vi "GOOP_LVClass_Item_OnCommand.vi"(10 "Command Tag":string, 11 "Object":u64) -> ()   [LabVIEW 2020]
uses:
  <resource>/Framework/Providers/Open_GDS/SubVIs/GOOP_ClassProviderClassType.ctl
  <resource>/Framework/Providers/Open_GDS/ClassProviders/Provider_BaseClassInterface/ClassWriter_class/ClassWriter.lvclass
  <resource>/Framework/Providers/Open_GDS/ClassProviders/Common/ScriptingFunctions/Scripting_ConnectorPanePatternType.ctl
  <resource>/Framework/Providers/Open_GDS/SubVIs/GOOP_UMLEditor_CallMainAction.ctl
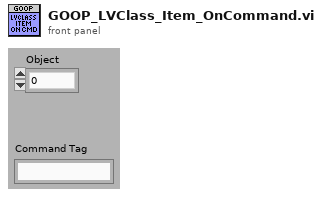
[diagram p1: front panel]
types:
  T1 = typedef "GOOP_ClassProviderClassType.ctl" = enum16{"ClassWriter", "ClassReader"}
  T2 = enum8{"No dynamic dispatch VIs", "Include nearest implementation", "Include all overrides"}
  T3 = typedef "GOOP_UMLEditor_CallMainAction.ctl" = enum16{"OpenUmlEditor", "ReverseEngineering:WholeProject", "ReverseEngineering:OneClass", "ReverseEngineering:OneVI", "ShowInStateDiagram:OneVI", "OpenUMLFile"}
  T4 = typedef "ClassWriter.lvclass/CreateMethodData.ctl" = cluster{"MethodName":string, "RelativeMethodPath":path, "MethodDescription":string, "Scope/Visibility":T5, "MethodTemplateName":string, "IconOut":u8[][], "RelativeProjectClassPath":string, "OpenViAfterCreation":bool, "DynamicDispatchVi":bool, "ExtraCreateParameters":variant, "MustOverride":bool, "MustCallParent":bool, "IconDetails":T6, "AF-Option":variant, "TemplatePath":path}
  T5 = typedef "GOOP300_MethodScopeType.ctl" = enum16{"Use Parent Folder Scope", "Public", "Protected", "Private", "Community"}
  T6 = typedef "ClassWriterNative.lvclass/IconDetails.ctl" = cluster{"IconSize":T7, "ImageRows(32)":i32, "ConnectorPaneHeight":i32[]}
  T7 = typedef "ClassWriterNative.lvclass/IconSize.ctl" = enum16{"Full", "1 c-term high", "2 c-term high", "3 c-term high"}
  T8 = typedef "AddDesignPatternData.ctl" = cluster{"Type":string, "ID":string, "Version":string, "VIPath":path, "Name":string, "Data":variant}
  T9 = typedef "ClassWriter.lvclass/CreateClassData.ctl" = cluster{"ClassName":string, "ClassFolder":path, "ClassDescription":string, "ClassTemplateOptions":string, "BaseClass(ProjectStringPath or LvClassFilePath)":variant, "ExtraCreateParameters":variant, "FolderSuffix":string}
  T10 = typedef "ClassWriter.lvclass/InterfacesToImplement.ctl" = cluster{"InterfacePath":path[], "CreateMethods":bool, "MethodsPerInterface(Empty=>All)":cluster{"Methods":string[]}[]}
  T11 = typedef "Scripting_ConnectorPanePatternType.ctl" = u16
  T12 = typedef "GDSLvCLass_ClassSettingsType.ctl" = cluster{"ClassProviderName":string, "ClassTemplateUsed":string, "ClassTemplateVersion":string, "ClassDescription":string, "PlugIns":T13[], "ConnectorPanePattern":string}
  T13 = typedef "GDSLvClass_PlugIn.ctl" = cluster{"Type":T14, "ID":string, "Version":string, "Path":path, "Name":string, "Data":variant}
  T14 = typedef "GDSLvClass_PlugInTypes.ctl" = enum16{"DesignPattern", "MethodTypes"}
  T15 = enum32{"invalid scope", "public", "private", "protected", "community"}
  T16 = typedef "ItemRef.ctl" = u64
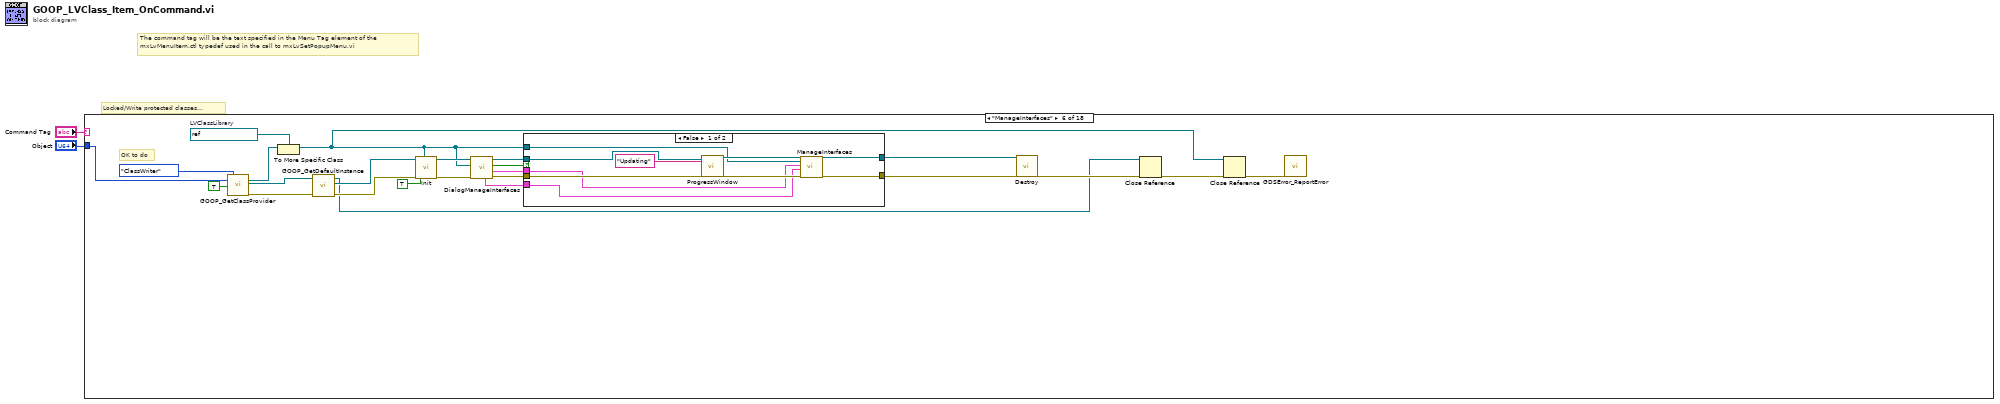
[diagram p0: block diagram]
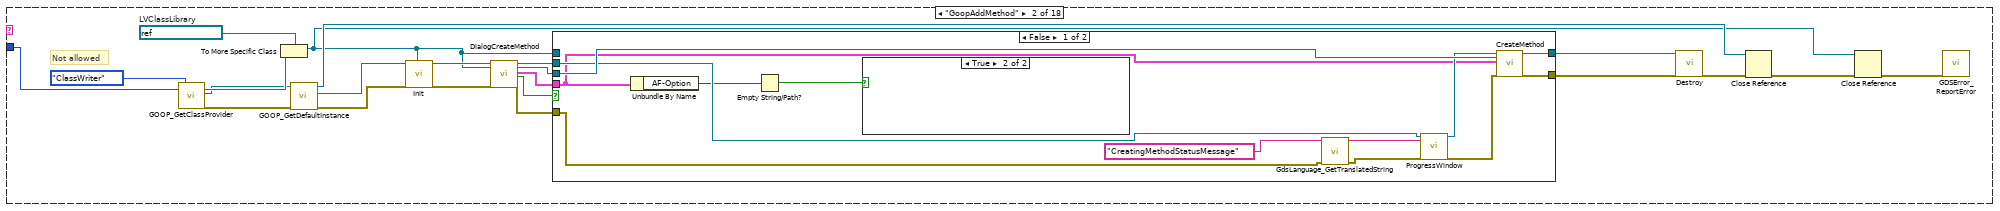
[diagram p3: hidden frame]
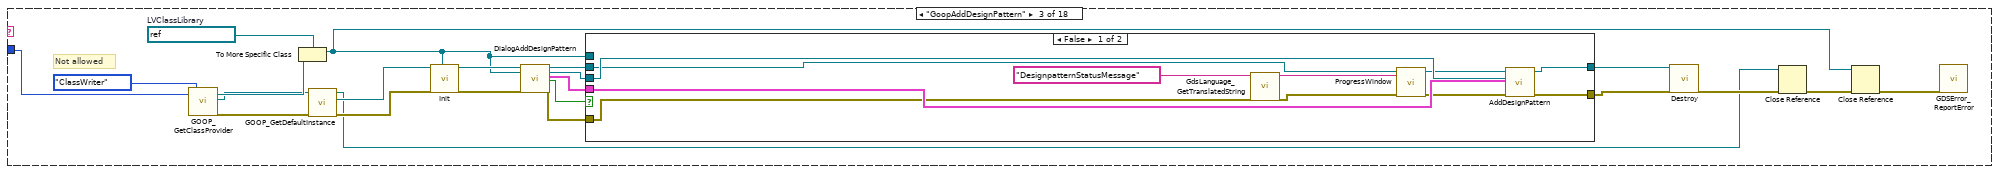
[diagram p6: hidden frame]
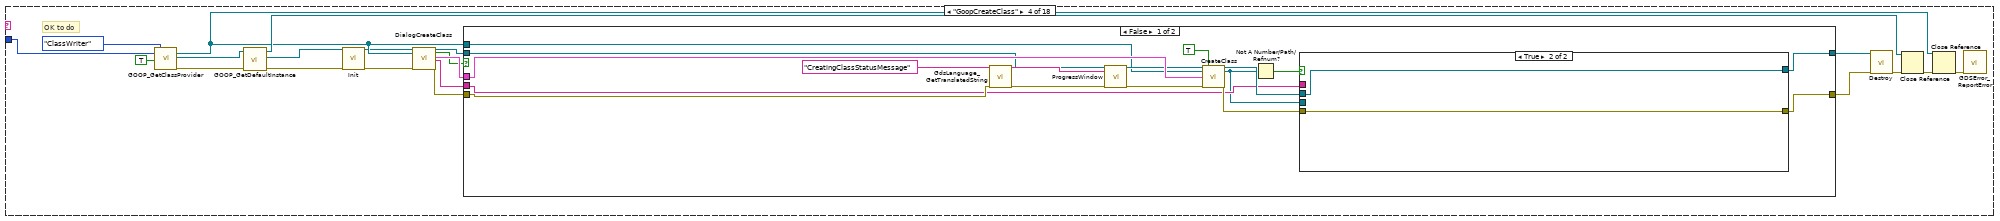
[diagram p8: hidden frame]
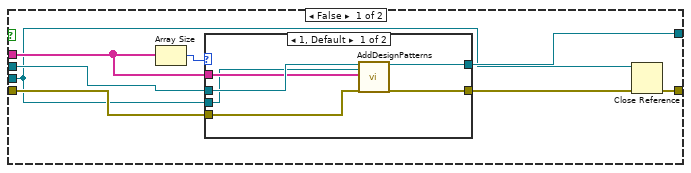
[diagram p9: hidden frame]
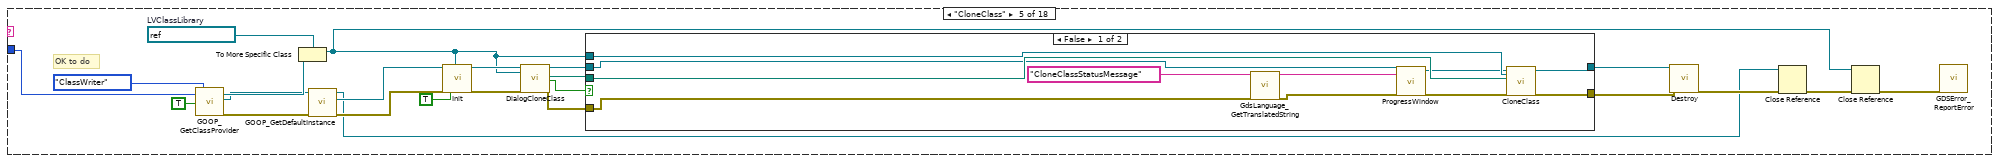
[diagram p12: hidden frame]
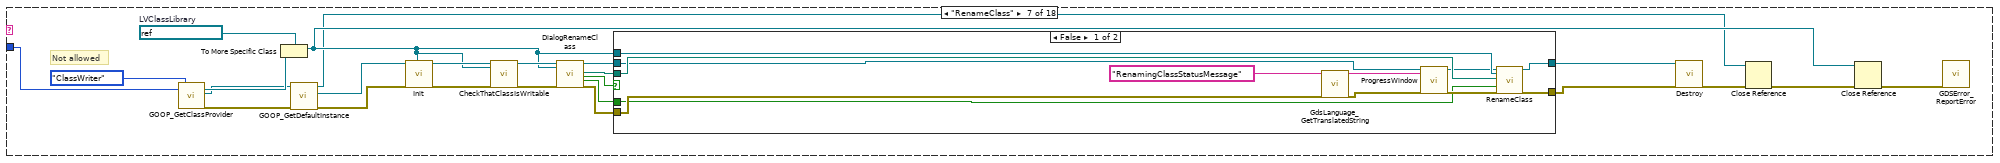
[diagram p15: hidden frame]
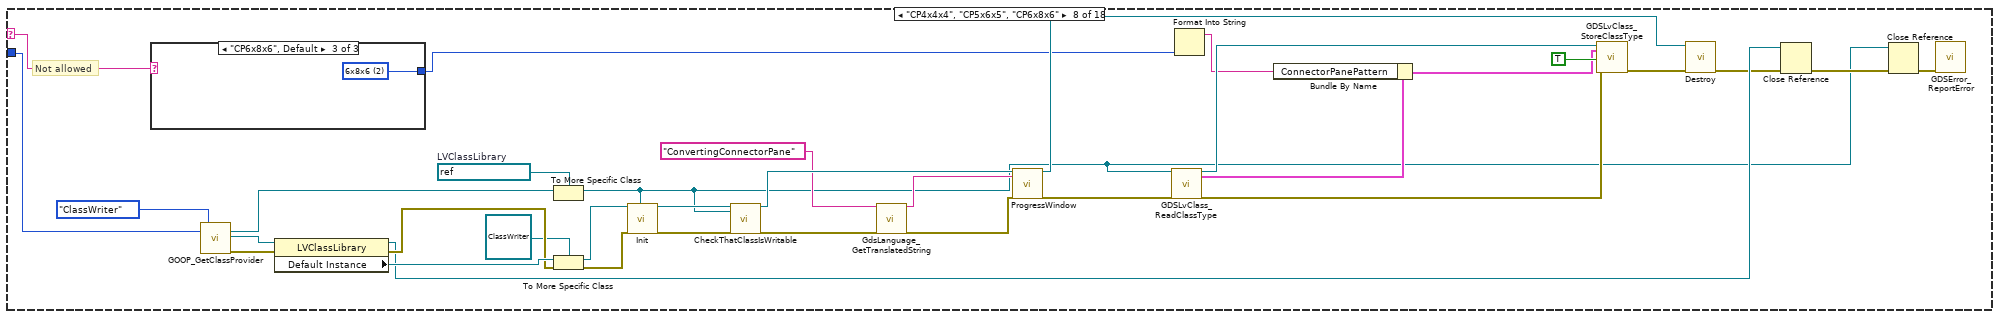
[diagram p17: hidden frame]
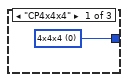
[diagram p18: hidden frame]
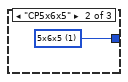
[diagram p19: hidden frame]
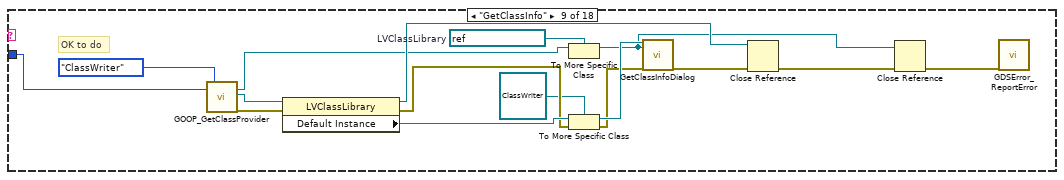
[diagram p20: hidden frame]
diagram:
  # "Locked/Write protected classes..."
  # "The command tag will be the text specified in the Menu Tag element of the \nmxLvMenuItem.ctl typedef used in the call to mxLvSetPopupMenu.vi"
  n1 = case shown="\"ManageInterfaces\"" "Command Tag" {
    selector: "Command Tag" -> [_ _ _ _ _ _ _ w243 _ _ _ _ _ _ w433 _ _ _]
    tunnel: "Object" -> [_ w24 w61 w95 w142 w185 w217 w263 w295 w296 w317 w324 w362 w381 w434 w463 w480 w527]
    frame "False" {
    }
    frame "GoopAddMethod" {
      w16 = refnum<vi> refnum  # LVClassLibrary
      # "Not allowed"
      n2 = call <resource>:"GOOP_GetClassProvider.vi"("New Item Parent/Object"=w24, "ProviderClassType"=GOOP_ClassProviderClassType."ClassWriter") -> ("ProjectItem"=w17:refnum<vi>, "LVClass.Open"=w5:refnum<vi>, "error out"=w4:errorcluster)  [unwired: 15 in]
      n3 = To More Specific Class(target class=w16, reference=w17) -> (specific class reference=w3:refnum<vi>)  [unwired: 1 in, 1 out]
      n4 = call <resource>:"GOOP_GetDefaultInstance.vi"("error in"=w4, "LVClassIn"=w5) -> ("error out"=w8:errorcluster, "ClassWriter.lvclass"=w7:refnum<class "ClassWriter.lvclass">, "LVClassOut"=w6:refnum<vi>)  [unwired: 7 in]
      n5 = call-dynamic "Init.vi"("ClassWriter in"=w7, "error in (no error)"=w8, "LVClassLibrary Refnum"=w3) -> ("ClassWriter out"=w9:refnum<class "ClassWriter.lvclass">, "error out"=w10:errorcluster)  [unwired: 15 in]
      n6 = call-dynamic "DialogCreateMethod.vi"("ClassWriter in"=w9, "ClassItemRefIn"=w3, "error in (no error)"=w10) -> ("ClassWriter out"=w20:refnum<class "ClassWriter.lvclass">, "ClassItemRefOut"=w19:refnum<vi>, "CreateMethodData"=w15:T4, "Cancelled"=w14:bool, "error out"=w18:errorcluster)  [unwired: 12 in]
      n7 = case shown="False" w14 {
        tunnel: w20 -> [w30 w38]
        tunnel: w19 -> [w37 _]
        tunnel: w18 -> [w32 w39]
        tunnel: w3 -> [_ _]
        tunnel: [w36 w39] -> w13
        tunnel: w15 -> [w27 _]
        tunnel: [w28 w38] -> w12
        frame False {
          n8 = Unbundle By Name(w27) -> ("AF-Option"=w26:variant)
          n9 = Empty String/Path?(string/path=w26) -> (empty?=w25:bool)
          n10 = case shown="True" w25 {
            frame False {
            }
            frame True {
            }
          }
          n11 = call <resource>:"GdsLanguage_GetTranslatedString.vi"("StringID(s)"="CreatingMethodStatusMessage" ("Message(Exit)"), "error in (no error)"=w32) -> ("FirstStringOut"=w35:string, "error out"=w34:errorcluster)  [unwired: 14 in, 2 out]
          n12 = call-dynamic "ProgressWindow.vi"("ClassWriter in"=w30, "Message(Exit)"=w35, "error in (no error)"=w34) -> ("ClassWriter out"=w29:refnum<class "ClassWriter.lvclass">, "error out"=w31:errorcluster)  [unwired: 15 in]
          n13 = call-dynamic "CreateMethod.vi"("ClassWriter.lvclass"=w29, "ClassItemRefIn"=w37, "CreateMethodData"=w27, "error in (no error)"=w31) -> ("ClassWriter.lvclass"=w28:refnum<class "ClassWriter.lvclass">, "error out"=w36:errorcluster)  [unwired: 12 in, 2 out]
        }
        frame True {
        }
      }
      n14 = call-dynamic "Destroy.vi"("ClassWriter.lvclass"=w12, "error in (no error)"=w13) -> ("error out"=w11:errorcluster)  [unwired: 17 in]
      n15 = Close Reference(reference=w6, error in (no error)=w11) -> (error out=w23:errorcluster)
      n16 = Close Reference(reference=w3, error in (no error)=w23) -> (error out=w22:errorcluster)
      n17 = call <resource>:"GDSError_ReportError.vi"("error in (no error)"=w22) -> ()  [unwired: 18 in, 1 out]
    }
    frame "GoopAddDesignPattern" {
      w53 = refnum<vi> refnum  # LVClassLibrary
      # "Not allowed"
      n18 = call <resource>:"GOOP_GetClassProvider.vi"("New Item Parent/Object"=w61, "ProviderClassType"=GOOP_ClassProviderClassType."ClassWriter") -> ("ProjectItem"=w54:refnum<vi>, "LVClass.Open"=w42:refnum<vi>, "error out"=w41:errorcluster)  [unwired: 15 in]
      n19 = To More Specific Class(target class=w53, reference=w54) -> (specific class reference=w40:refnum<vi>)  [unwired: 1 in, 1 out]
      n20 = call <resource>:"GOOP_GetDefaultInstance.vi"("error in"=w41, "LVClassIn"=w42) -> ("error out"=w45:errorcluster, "ClassWriter.lvclass"=w44:refnum<class "ClassWriter.lvclass">, "LVClassOut"=w43:refnum<vi>)  [unwired: 7 in]
      n21 = call-dynamic "Init.vi"("ClassWriter in"=w44, "error in (no error)"=w45, "LVClassLibrary Refnum"=w40) -> ("ClassWriter out"=w46:refnum<class "ClassWriter.lvclass">, "error out"=w47:errorcluster)  [unwired: 15 in]
      n22 = call-dynamic "DialogAddDesignPattern.vi"("ClassWriter in"=w46, "ClassItemRefIn"=w40, "error in (no error)"=w47) -> ("ClassWriter out"=w57:refnum<class "ClassWriter.lvclass">, "ClassItemRefOut"=w56:refnum<vi>, "CreateMethodData"=w52:T8, "Cancelled"=w51:bool, "error out"=w55:errorcluster)  [unwired: 12 in]
      n23 = case shown="False" w51 {
        tunnel: w57 -> [w64 w73]
        tunnel: w56 -> [w72 _]
        tunnel: w55 -> [w66 w74]
        tunnel: w40 -> [_ _]
        tunnel: [w70 w74] -> w50
        tunnel: w52 -> [w71 _]
        tunnel: [w62 w73] -> w49
        frame False {
          n24 = call <resource>:"GdsLanguage_GetTranslatedString.vi"("StringID(s)"="DesignpatternStatusMessage" ("Message(Exit)"), "error in (no error)"=w66) -> ("FirstStringOut"=w69:string, "error out"=w68:errorcluster)  [unwired: 14 in, 2 out]
          n25 = call-dynamic "ProgressWindow.vi"("ClassWriter in"=w64, "Message(Exit)"=w69, "error in (no error)"=w68) -> ("ClassWriter out"=w63:refnum<class "ClassWriter.lvclass">, "error out"=w65:errorcluster)  [unwired: 15 in]
          n26 = call-dynamic "AddDesignPattern.vi"("ClassWriter.lvclass"=w63, "ClassItemRefIn"=w72, "AddDesignPatternData"=w71, "error in (no error)"=w65) -> ("ClassWriter.lvclass"=w62:refnum<class "ClassWriter.lvclass">, "error out"=w70:errorcluster)  [unwired: 13 in, 1 out]
        }
        frame True {
        }
      }
      n27 = call-dynamic "Destroy.vi"("ClassWriter.lvclass"=w49, "error in (no error)"=w50) -> ("error out"=w48:errorcluster)  [unwired: 17 in]
      n28 = Close Reference(reference=w43, error in (no error)=w48) -> (error out=w60:errorcluster)
      n29 = Close Reference(reference=w40, error in (no error)=w60) -> (error out=w59:errorcluster)
      n30 = call <resource>:"GDSError_ReportError.vi"("error in (no error)"=w59) -> ()  [unwired: 18 in, 1 out]
    }
    frame "GoopCreateClass" {
      # "OK to do"
      n31 = call <resource>:"GOOP_GetClassProvider.vi"("New Item Parent/Object"=w95, "CreateClass"=TRUE, "ProviderClassType"=GOOP_ClassProviderClassType."ClassWriter") -> ("ProjectItem"=w84:refnum<vi>, "LVClass.Open"=w92:refnum<vi>, "error out"=w91:errorcluster)  [unwired: 14 in]
      n32 = call <resource>:"GOOP_GetDefaultInstance.vi"("error in"=w91, "LVClassIn"=w92) -> ("error out"=w76:errorcluster, "ClassWriter.lvclass"=w77:refnum<class "ClassWriter.lvclass">, "LVClassOut"=w87:refnum<vi>)  [unwired: 7 in]
      n33 = call-dynamic "Init.vi"("ClassWriter in"=w77, "error in (no error)"=w76) -> ("ClassWriter out"=w79:refnum<class "ClassWriter.lvclass">, "error out"=w78:errorcluster)  [unwired: 16 in]
      n34 = call-dynamic "DialogCreateClass.vi"("ClassWriter in"=w79, "ProjectItem Refnum"=w84, "error in (no error)"=w78) -> ("ClassWriter out"=w89:refnum<class "ClassWriter.lvclass">, "Cancelled"=w85:bool, "CreateClassData"=w86:T9, "DesignPatternsToAddAfterCreation"=w75:string[], "error out"=w88:errorcluster)  [unwired: 10 in, 2 out]
      n35 = case shown="False" w85 {
        tunnel: w89 -> [w107 w131]
        tunnel: w88 -> [w108 w132]
        tunnel: w84 -> [w100 _]
        tunnel: [w98 w132] -> w83
        tunnel: w86 -> [w112 _]
        tunnel: [w102 w131] -> w81
        tunnel: w75 -> [w101 _]
        frame False {
          n36 = call <resource>:"GdsLanguage_GetTranslatedString.vi"("StringID(s)"="CreatingClassStatusMessage" ("Message(Exit)"), "error in (no error)"=w108) -> ("FirstStringOut"=w109:string, "error out"=w110:errorcluster)  [unwired: 14 in, 2 out]
          n37 = call-dynamic "ProgressWindow.vi"("ClassWriter in"=w107, "Message(Exit)"=w109, "error in (no error)"=w110) -> ("ClassWriter out"=w106:refnum<class "ClassWriter.lvclass">, "error out"=w105:errorcluster)  [unwired: 15 in]
          n38 = call-dynamic "CreateClass.vi"("ClassWriter.lvclass"=w106, "ProjectTreePosition(String or Project Item Ref)"=w100, "CreateClassData"=w112, "error in (no error)"=w105, "KeepLvClassRefOpen(False)"=TRUE) -> ("ClassWriter.lvclass"=w104:refnum<class "ClassWriter.lvclass">, "LVClassLibraryRefnum"=w97:refnum<vi>, "error out"=w103:errorcluster)  [unwired: 11 in, 1 out]
          n39 = Not A Number/Path/Refnum?(number/path/refnum=w97) -> (NaN/Path/Refnum?=w96:bool)
          n40 = case shown="True" w96 {
            tunnel: w104 -> [w119 w130]
            tunnel: w103 -> [w118 w129]
            tunnel: [w117 w130] -> w102
            tunnel: w101 -> [w116 _]
            tunnel: [w114 w129] -> w98
            tunnel: w97 -> [w113 _]
            frame False {
              n41 = Array Size(array=w116) -> (size(s)=w120:i32)
              n42 = case shown="1, Default" w120 {
                tunnel: w119 -> [w126 w128]
                tunnel: w118 -> [w125 w127]
                tunnel: [w124 w127] -> w115
                tunnel: [w123 w128] -> w117
                tunnel: w116 -> [w122 _]
                tunnel: w113 -> [w121 _]
                frame 1, Default {
                  n43 = call-dynamic "AddDesignPatterns.vi"("ClassWriterNative"=w126, "ClassItemRefIn"=w121, "DesignPatterns"=w122, "error in (no error)"=w125) -> ("ClassWriterNative"=w123:refnum<class "ClassWriter.lvclass">, "error out"=w124:errorcluster)  [unwired: 12 in, 2 out]
                }
                frame 0 {
                }
              }
              n44 = Close Reference(reference=w113, error in (no error)=w115) -> (error out=w114:errorcluster)
            }
            frame True {
            }
          }
        }
        frame True {
        }
      }
      n45 = call-dynamic "Destroy.vi"("ClassWriter.lvclass"=w81, "error in (no error)"=w83) -> ("error out"=w82:errorcluster)  [unwired: 17 in]
      n46 = Close Reference(reference=w87, error in (no error)=w82) -> (error out=w94:errorcluster)
      n47 = Close Reference(reference=w84, error in (no error)=w94) -> (error out=w93:errorcluster)
      n48 = call <resource>:"GDSError_ReportError.vi"("error in (no error)"=w93) -> ()  [unwired: 18 in, 1 out]
    }
    frame "CloneClass" {
      w152 = refnum<vi> refnum  # LVClassLibrary
      # "OK to do"
      n49 = call <resource>:"GOOP_GetClassProvider.vi"("New Item Parent/Object"=w142, "CreateClass"=TRUE, "ProviderClassType"=GOOP_ClassProviderClassType."ClassWriter") -> ("ProjectItem"=w153:refnum<vi>, "LVClass.Open"=w139:refnum<vi>, "error out"=w140:errorcluster)  [unwired: 14 in]
      n50 = To More Specific Class(target class=w152, reference=w153) -> (specific class reference=w133:refnum<vi>)  [unwired: 1 in, 1 out]
      n51 = call <resource>:"GOOP_GetDefaultInstance.vi"("error in"=w140, "LVClassIn"=w139) -> ("error out"=w137:errorcluster, "ClassWriter.lvclass"=w138:refnum<class "ClassWriter.lvclass">, "LVClassOut"=w136:refnum<vi>)  [unwired: 7 in]
      n52 = call-dynamic "Init.vi"("ClassWriter in"=w138, "error in (no error)"=w137, "ClassFileMayBeReadOnly(False)"=TRUE, "LVClassLibrary Refnum"=w133) -> ("ClassWriter out"=w145:refnum<class "ClassWriter.lvclass">, "error out"=w144:errorcluster)  [unwired: 14 in]
      n53 = call-dynamic "DialogCloneClass.vi"("ClassWriter.lvclass"=w145, "ClassItemRefIn"=w133, "error in (no error)"=w144) -> ("ClassWriter.lvclassOut"=w150:refnum<class "ClassWriter.lvclass">, "NewClassPath"=w146:path, "Cancelled"=w147:bool, "error out"=w149:errorcluster)  [unwired: 12 in, 1 out]
      n54 = case shown="False" w147 {
        tunnel: w150 -> [w158 w167]
        tunnel: w149 -> [w159 w168]
        tunnel: [w163 w168] -> w148
        tunnel: w133 -> [w166 _]
        tunnel: w146 -> [w165 _]
        tunnel: [w164 w167] -> w143
        frame False {
          n55 = call <resource>:"GdsLanguage_GetTranslatedString.vi"("StringID(s)"="CloneClassStatusMessage" ("Message(Exit)"), "error in (no error)"=w159) -> ("FirstStringOut"=w160:string, "error out"=w161:errorcluster)  [unwired: 14 in, 2 out]
          n56 = call-dynamic "ProgressWindow.vi"("ClassWriter in"=w158, "Message(Exit)"=w160, "error in (no error)"=w161) -> ("ClassWriter out"=w157:refnum<class "ClassWriter.lvclass">, "error out"=w156:errorcluster)  [unwired: 15 in]
          n57 = call-dynamic "CloneClass.vi"("ClassWriter.lvclass"=w157, "ClassRef"=w166, "NewClassPath"=w165, "error in (no error)"=w156) -> ("ClassWriter.lvclass"=w164:refnum<class "ClassWriter.lvclass">, "error out"=w163:errorcluster)  [unwired: 13 in, 1 out]
        }
        frame True {
        }
      }
      n58 = call-dynamic "Destroy.vi"("ClassWriter.lvclass"=w143, "error in (no error)"=w148) -> ("error out"=w151:errorcluster)  [unwired: 17 in]
      n59 = Close Reference(reference=w136, error in (no error)=w151) -> (error out=w155:errorcluster)
      n60 = Close Reference(reference=w133, error in (no error)=w155) -> (error out=w141:errorcluster)
      n61 = call <resource>:"GDSError_ReportError.vi"("error in (no error)"=w141) -> ()  [unwired: 18 in, 1 out]
    }
    frame "ManageInterfaces" {
      w189 = refnum<vi> refnum  # LVClassLibrary
      # "OK to do"
      n62 = call <resource>:"GOOP_GetClassProvider.vi"("New Item Parent/Object"=w185, "CreateClass"=TRUE, "ProviderClassType"=GOOP_ClassProviderClassType."ClassWriter") -> ("ProjectItem"=w190:refnum<vi>, "LVClass.Open"=w182:refnum<vi>, "error out"=w183:errorcluster)  [unwired: 14 in]
      n63 = To More Specific Class(target class=w189, reference=w190) -> (specific class reference=w171:refnum<vi>)  [unwired: 1 in, 1 out]
      n64 = call <resource>:"GOOP_GetDefaultInstance.vi"("error in"=w183, "LVClassIn"=w182) -> ("error out"=w180:errorcluster, "ClassWriter.lvclass"=w181:refnum<class "ClassWriter.lvclass">, "LVClassOut"=w179:refnum<vi>)  [unwired: 7 in]
      n65 = call-dynamic "Init.vi"("ClassWriter in"=w181, "error in (no error)"=w180, "ClassFileMayBeReadOnly(False)"=TRUE, "LVClassLibrary Refnum"=w171) -> ("ClassWriter out"=w176:refnum<class "ClassWriter.lvclass">, "error out"=w175:errorcluster)  [unwired: 14 in]
      n66 = call-dynamic "DialogManageInterfaces.vi"("error in (no error)"=w175, "ClassItemRefIn"=w171, "ClassWriterIn"=w176) -> ("error out"=w173:errorcluster, "InterfaceToAdd"=w170:T10, "Cancelled"=w174:bool, "ClassWriterOut"=w172:refnum<class "ClassWriter.lvclass">, "InterfaceToRemove(CreateMethod=>RemoveMethods)"=w169:T10)  [unwired: 4 in]
      n67 = case shown="False" w174 {
        tunnel: w172 -> [w202 w203]
        tunnel: w173 -> [w200 w204]
        tunnel: [w197 w204] -> w187
        tunnel: w171 -> [w195 _]
        tunnel: [w196 w203] -> w186
        tunnel: w170 -> [w194 _]
        tunnel: w169 -> [w193 _]
        frame False {
          n68 = call-dynamic "ProgressWindow.vi"("ClassWriter in"=w202, "Message(Exit)"="Updating", "error in (no error)"=w200) -> ("ClassWriter out"=w199:refnum<class "ClassWriter.lvclass">, "error out"=w198:errorcluster)  [unwired: 15 in]
          n69 = call-dynamic "ManageInterfaces.vi"("ClassWriter.lvclass"=w199, "ClassRef"=w195, "InterfaceToAdd"=w194, "InterfaceToRemove(CreateMethod=>RemoveMethods)"=w193, "error in (no error)"=w198) -> ("ClassWriter.lvclass"=w196:refnum<class "ClassWriter.lvclass">, "error out"=w197:errorcluster)  [unwired: 13 in]
        }
        frame True {
        }
      }
      n70 = call-dynamic "Destroy.vi"("ClassWriter.lvclass"=w186, "error in (no error)"=w187) -> ("error out"=w188:errorcluster)  [unwired: 17 in]
      n71 = Close Reference(reference=w179, error in (no error)=w188) -> (error out=w192:errorcluster)
      n72 = Close Reference(reference=w171, error in (no error)=w192) -> (error out=w184:errorcluster)
      n73 = call <resource>:"GDSError_ReportError.vi"("error in (no error)"=w184) -> ()  [unwired: 18 in, 1 out]
    }
    frame "RenameClass" {
      w225 = refnum<vi> refnum  # LVClassLibrary
      # "Not allowed"
      n74 = call <resource>:"GOOP_GetClassProvider.vi"("New Item Parent/Object"=w217, "ProviderClassType"=GOOP_ClassProviderClassType."ClassWriter") -> ("ProjectItem"=w226:refnum<vi>, "LVClass.Open"=w208:refnum<vi>, "error out"=w209:errorcluster)  [unwired: 15 in]
      n75 = To More Specific Class(target class=w225, reference=w226) -> (specific class reference=w211:refnum<vi>)  [unwired: 1 in, 1 out]
      n76 = call <resource>:"GOOP_GetDefaultInstance.vi"("error in"=w209, "LVClassIn"=w208) -> ("error out"=w206:errorcluster, "ClassWriter.lvclass"=w207:refnum<class "ClassWriter.lvclass">, "LVClassOut"=w205:refnum<vi>)  [unwired: 7 in]
      n77 = call-dynamic "Init.vi"("ClassWriter in"=w207, "error in (no error)"=w206, "LVClassLibrary Refnum"=w211) -> ("ClassWriter out"=w215:refnum<class "ClassWriter.lvclass">, "error out"=w214:errorcluster)  [unwired: 15 in]
      n78 = call <resource>:"CheckThatClassIsWritable.vi"("ClassWriter in"=w215, "Library Refnum"=w211, "error in (no error)"=w214) -> ("ClassWriter out"=w213:refnum<class "ClassWriter.lvclass">, "error out"=w212:errorcluster)  [unwired: 15 in]
      n79 = call-dynamic "DialogRenameClass.vi"("ClassWriter.lvclass"=w213, "ClassItemRefIn"=w211, "error in (no error)"=w212) -> ("ClassWriter.lvclassOut"=w223:refnum<class "ClassWriter.lvclass">, "NewClassPath"=w219:path, "Cancelled"=w220:bool, "RelinkWholeProject"=w210:bool, "error out"=w222:errorcluster)  [unwired: 11 in, 1 out]
      n80 = case shown="False" w220 {
        tunnel: w223 -> [w236 w241]
        tunnel: w222 -> [w233 w242]
        tunnel: [w237 w242] -> w221
        tunnel: w211 -> [w240 _]
        tunnel: w219 -> [w239 _]
        tunnel: [w238 w241] -> w218
        tunnel: w210 -> [w229 _]
        frame False {
          n81 = call <resource>:"GdsLanguage_GetTranslatedString.vi"("StringID(s)"="RenamingClassStatusMessage" ("Message(Exit)"), "error in (no error)"=w233) -> ("FirstStringOut"=w230:string, "error out"=w232:errorcluster)  [unwired: 14 in, 2 out]
          n82 = call-dynamic "ProgressWindow.vi"("ClassWriter in"=w236, "Message(Exit)"=w230, "error in (no error)"=w232) -> ("ClassWriter out"=w235:refnum<class "ClassWriter.lvclass">, "error out"=w234:errorcluster)  [unwired: 15 in]
          n83 = call-dynamic "RenameClass.vi"("ClassWriter.lvclass"=w235, "ClassRef"=w240, "NewClassPath"=w239, "RelinkWholeProject"=w229, "error in (no error)"=w234) -> ("ClassWriter.lvclass"=w238:refnum<class "ClassWriter.lvclass">, "error out"=w237:errorcluster)  [unwired: 13 in]
        }
        frame True {
        }
      }
      n84 = call-dynamic "Destroy.vi"("ClassWriter.lvclass"=w218, "error in (no error)"=w221) -> ("error out"=w224:errorcluster)  [unwired: 17 in]
      n85 = Close Reference(reference=w205, error in (no error)=w224) -> (error out=w228:errorcluster)
      n86 = Close Reference(reference=w211, error in (no error)=w228) -> (error out=w216:errorcluster)
      n87 = call <resource>:"GDSError_ReportError.vi"("error in (no error)"=w216) -> ()  [unwired: 18 in, 1 out]
    }
    frame "CP4x4x4", "CP5x6x5", "CP6x8x6" {
      w269 = refnum<vi> refnum  # LVClassLibrary
      # "Not allowed"
      n88 = case shown="\"CP6x8x6\", Default" w243 {
        tunnel: [w277 w278 w279] -> w245
        frame "CP4x4x4" {
          w277 = T11 0 items=["4x4x4", "5x6x5", "6x8x6"] ("Pattern")
        }
        frame "CP5x6x5" {
          w278 = T11 1 items=["4x4x4", "5x6x5", "6x8x6"] ("Pattern")
        }
        frame "CP6x8x6", Default {
          w279 = T11 2 items=["4x4x4", "5x6x5", "6x8x6"] ("Pattern")
        }
      }
      n89 = call <resource>:"GOOP_GetClassProvider.vi"("New Item Parent/Object"=w263, "ProviderClassType"=GOOP_ClassProviderClassType."ClassWriter") -> ("ProjectItem"=w270:refnum<vi>, "LVClass.Open"=w268:refnum<vi>, "error out"=w273:errorcluster)  [unwired: 15 in]
      n90 = property class="LVClassLibrary"(reference=w268, error in=w273) -> (reference out=w271:refnum<vi>, error out=w275:errorcluster, "Default Instance"=w276:refnum<class>)
      n91 = To More Specific Class(target class=w269, reference=w270) -> (specific class reference=w249:refnum<vi>)  [unwired: 1 in, 1 out]
      n92 = To More Specific Class(target class=refnum<class "ClassWriter.lvclass"> refnum ("ClassWriter.lvclass"), reference=w276, error in=w275) -> (specific class reference=w264:refnum<class "ClassWriter.lvclass">, error out=w265:errorcluster)
      n93 = call-dynamic "Init.vi"("ClassWriter in"=w264, "error in (no error)"=w265, "LVClassLibrary Refnum"=w249) -> ("ClassWriter out"=w261:refnum<class "ClassWriter.lvclass">, "error out"=w260:errorcluster)  [unwired: 15 in]
      n94 = call <resource>:"CheckThatClassIsWritable.vi"("ClassWriter in"=w261, "Library Refnum"=w249, "error in (no error)"=w260) -> ("ClassWriter out"=w258:refnum<class "ClassWriter.lvclass">, "error out"=w259:errorcluster)  [unwired: 15 in]
      n95 = call <resource>:"GdsLanguage_GetTranslatedString.vi"("StringID(s)"="ConvertingConnectorPane" ("Message(Exit)"), "error in (no error)"=w259) -> ("FirstStringOut"=w255:string, "error out"=w257:errorcluster)  [unwired: 14 in, 2 out]
      n96 = call-dynamic "ProgressWindow.vi"("ClassWriter in"=w258, "Message(Exit)"=w255, "error in (no error)"=w257) -> ("ClassWriter out"=w254:refnum<class "ClassWriter.lvclass">, "error out"=w253:errorcluster)  [unwired: 15 in]
      n97 = call <resource>:"GDSLvClass_ReadClassType.vi"("Class Refnum In"=w249, "error in (no error)"=w253) -> ("Class Refnum Out"=w252:refnum<vi>, "ClassSettings"=w251:T12, "error out"=w250:errorcluster)  [unwired: 15 in]
      n98 = Format Into String(w245) -> (resulting string=w244:string)  [unwired: 3 in, 1 out]
      n99 = Bundle By Name(cluster=w251, "ConnectorPanePattern"=w244) -> (w246:T12)
      n100 = call <resource>:"GDSLvClass_StoreClassType.vi"("Class Refnum In"=w252, "ClassSettings"=w246, "CheckAndFixConnectorPaneType(False)"=TRUE, "error in (no error)"=w250) -> ("error out"=w248:errorcluster)  [unwired: 14 in, 1 out]
      n101 = call-dynamic "Destroy.vi"("ClassWriter.lvclass"=w254, "error in (no error)"=w248) -> ("error out"=w267:errorcluster)  [unwired: 17 in]
      n102 = Close Reference(reference=w271, error in (no error)=w267) -> (error out=w274:errorcluster)
      n103 = Close Reference(reference=w249, error in (no error)=w274) -> (error out=w262:errorcluster)
      n104 = call <resource>:"GDSError_ReportError.vi"("error in (no error)"=w262) -> ()  [unwired: 18 in, 1 out]
    }
    frame "GetClassInfo" {
      w284 = refnum<vi> refnum  # LVClassLibrary
      # "OK to do"
      n105 = call <resource>:"GOOP_GetClassProvider.vi"("New Item Parent/Object"=w295, "ProviderClassType"=GOOP_ClassProviderClassType."ClassWriter") -> ("ProjectItem"=w285:refnum<vi>, "LVClass.Open"=w290:refnum<vi>, "error out"=w289:errorcluster)  [unwired: 15 in]
      n106 = property class="LVClassLibrary"(reference=w290, error in=w289) -> (reference out=w287:refnum<vi>, error out=w293:errorcluster, "Default Instance"=w294:refnum<class>)
      n107 = To More Specific Class(target class=w284, reference=w285) -> (specific class reference=w280:refnum<vi>)  [unwired: 1 in, 1 out]
      n108 = To More Specific Class(target class=refnum<class "ClassWriter.lvclass"> refnum ("ClassWriter.lvclass"), reference=w294, error in=w293) -> (specific class reference=w283:refnum<class "ClassWriter.lvclass">, error out=w282:errorcluster)
      n109 = call-dynamic "GetClassInfoDialog.vi"("ClassWriter in"=w283, "ClassItemRefIn"=w280, "error in (no error)"=w282) -> ("error out"=w281:errorcluster)  [unwired: 15 in, 1 out]
      n110 = Close Reference(reference=w287, error in (no error)=w281) -> (error out=w292:errorcluster)
      n111 = Close Reference(reference=w280, error in (no error)=w292) -> (error out=w291:errorcluster)
      n112 = call <resource>:"GDSError_ReportError.vi"("error in (no error)"=w291) -> ()  [unwired: 18 in, 1 out]
    }
    frame "DebugClass" {
      w305 = refnum<vi> refnum  # LVClassLibrary
      # "OK to do"
      n113 = call <resource>:"GOOP_GetClassProvider.vi"("New Item Parent/Object"=w296, "ProviderClassType"=GOOP_ClassProviderClassType."ClassWriter") -> ("ProjectItem"=w306:refnum<vi>, "LVClass.Open"=w304:refnum<vi>, "error out"=w297:errorcluster)  [unwired: 15 in]
      n114 = To More Specific Class(target class=w305, reference=w306, error in=w297) -> (specific class reference=w303:refnum<vi>, error out=w298:errorcluster)
      n115 = property class="LVClassLibrary"(reference=w303, error in=w298) -> (reference out=w302:refnum<vi>, error out=w299:errorcluster, "Name"=w301:string)
      n116 = call <resource>:"GOOP_StartObjectDebugger.vi"("ClassToOpen"=w301, "error in (no error)"=w299) -> ("error out"=w300:errorcluster)  [unwired: 17 in]
      n117 = Close Reference(reference=w304, error in (no error)=w300) -> (error out=w309:errorcluster)
      n118 = Close Reference(reference=w302, error in (no error)=w309) -> (error out=w308:errorcluster)
      n119 = call <resource>:"GDSError_ReportError.vi"("error in (no error)"=w308) -> ()  [unwired: 18 in, 1 out]
    }
    frame "GoopEditClassIcon" {
      w318 = refnum<vi> refnum  # LVClassLibrary
      # "Not allowed"
      n120 = call <resource>:"mxLvGetItemRef.vi"("Item"=w317) -> ("Item Refnum"=w316:refnum<vi>, "error out"=w311:errorcluster)  [unwired: 1 in, 1 out]
      n121 = To More Specific Class(target class=w318, reference=w316) -> (specific class reference=w310:refnum<vi>)  [unwired: 1 in, 1 out]
      n122 = call <resource>:"GOOP_CheckClassState.vi"("error in"=w311, "Library Refnum"=w310) -> ("error out"=w312:errorcluster)  [unwired: 9 in]
      n123 = call <resource>:"CheckThatClassIsWritable.vi"("Library Refnum"=w310, "error in (no error)"=w312) -> ("error out"=w313:errorcluster)  [unwired: 16 in, 1 out]
      n124 = call <resource>:"GDSLvIcon_DialogUpdateClass.vi"("ClassPath(FilePath/ProjectTreePath/LvCLassRef)"=w310, "error in (no error)"=w313) -> ("error out"=w315:errorcluster)  [unwired: 14 in, 3 out]
      n125 = Close Reference(reference=w310, error in (no error)=w315) -> (error out=w314:errorcluster)
      n126 = call <resource>:"GDSError_ReportError.vi"("error in (no error)"=w314) -> ()  [unwired: 18 in, 1 out]
    }
    frame "ClassTool" {
      w325 = refnum<vi> refnum  # LVClassLibrary
      # "Not allowed"
      n127 = call <resource>:"mxLvGetItemRef.vi"("Item"=w324) -> ("Item Refnum"=w323:refnum<vi>, "error out"=w321:errorcluster)  [unwired: 1 in, 1 out]
      n128 = To More Specific Class(target class=w325, reference=w323) -> (specific class reference=w320:refnum<vi>)  [unwired: 1 in, 1 out]
      n129 = call <resource>:"GOOP_ClassTool.vi"("ClassRef"=w320, "Error In"=w321) -> ("Error Out"=w319:errorcluster)  [unwired: 17 in]
      n130 = Close Reference(reference=w320, error in (no error)=w319) -> (error out=w322:errorcluster)
      n131 = call <resource>:"GDSError_ReportError.vi"("error in (no error)"=w322) -> ()  [unwired: 18 in, 1 out]
    }
    frame "UpdateMessageClass" {
      w363 = refnum<vi> refnum  # LVClassLibrary
      # "From Message Class Ref\nGet Actor method"
      # "Not allowed"
      n132 = call <resource>:"mxLvGetItemRef.vi"("Item"=w362) -> ("Item Refnum"=w361:refnum<vi>, "error out"=w337:errorcluster)  [unwired: 1 in, 1 out]
      n133 = call-dynamic "Init.vi"("ClassWriter in"=refnum<class "ClassWriter.lvclass"> refnum, "error in (no error)"=w337) -> ("ClassWriter out"=w331:refnum<class "ClassWriter.lvclass">, "error out"=w334:errorcluster)  [unwired: 16 in]
      n134 = call <resource>:"GdsLanguage_GetTranslatedString.vi"("StringID(s)"="UpdateMessageClass" ("Message(Exit)"), "error in (no error)"=w334) -> ("FirstStringOut"=w335:string, "error out"=w333:errorcluster)  [unwired: 14 in, 2 out]
      n135 = disable-structure shown="Enabled" {
        disable-tunnel: w335 -> [w368 _]
        disable-tunnel: [w367 w370] -> w328
        disable-tunnel: w333 -> [w366 w370]
        disable-tunnel: w331 -> [w365 w369]
        disable-tunnel: [w364 w369] -> w330
        frame Enabled {
          n136 = call-dynamic "ProgressWindow.vi"("ClassWriter in"=w365, "Message(Exit)"=w368, "error in (no error)"=w366) -> ("ClassWriter out"=w364:refnum<class "ClassWriter.lvclass">, "error out"=w367:errorcluster)  [unwired: 15 in]
        }
        frame Disabled {
        }
      }
      n137 = To More Specific Class(target class=w363, reference=w361) -> (specific class reference=w327:refnum<vi>)  [unwired: 1 in, 1 out]
      n138 = property class="LVClassLibrary"(reference=w327, error in=w328) -> (error out=w359:errorcluster, "Project"=w358:refnum<vi>, "Path"=w355:path)  [unwired: 1 out]
      n139 = property class="Project"(reference=w358, error in=w359) -> (error out=w348:errorcluster, "App Ref"=w357:refnum<vi>)  [unwired: 1 out]
      n140 = invoke class="LVClassLibrary" method="Get All Descendents"(reference=w327, error in=w348, "Type"="VI") -> (error out=w350:errorcluster, "All Descendents"=w342:refnum<vi>[])  [unwired: 4 in, 5 out]
      n141 = for {
        tunnel: w342 -> [w378] mode=indexing
        tunnel: [w374] -> w352
        shift-right: [w373] -> w351
        shift-left: w350 -> [w372]
        stop <- w371 stop-if-true
        n142 = property class="ProjectItem"(reference=w378, error in=w372) -> (reference out=w374:refnum<vi>, error out=w373:errorcluster, "Name"=w377:string)
        n143 = To Lower Case(string=w377) -> (all lower case string=w376:string)
        n144 = Equal?(x=w376, y="do.vi") -> (x = y?=w371:bool)
      }
      n145 = Strip Path(path=w355) -> (stripped path=w354:path)  [unwired: 1 out]
      n146 = property class="ProjectItem"(reference=w352, error in=w351) -> (error out=w346:errorcluster, "Reference"=w349:refnum<vi>)  [unwired: 1 out]
      n147 = invoke class="VI" method="Get VI Dependencies"(reference=w349, error in=w346, "Dynamic Dispatching?"=T2."Include nearest implementation") -> (reference out=w344:refnum<vi>, error out=w345:errorcluster, "Dependency Paths"=w341:path[])  [unwired: 16 in, 16 out]
      n148 = Close Reference(reference=w344, error in (no error)=w345) -> (error out=w343:errorcluster)
      n149 = Index Array(array=w341) -> (element=w340:path)  [unwired: 1 in]
      n150 = Close Reference(reference=w342, error in (no error)=w343) -> (error out=w339:errorcluster)
      n151 = call <resource>:"MM.vi"("AppInst"=w357, "ActorMethod"=w340, "ActorClassItemRef(Don't Delete)"=refnum<vi> refnum, "OnlyUpdate(if needed,False)"=TRUE ("OnlyUpdate(if needed)"), "Destination Path"=w354, "error in"=w339) -> ("error out"=w338:errorcluster)  [unwired: 13 in]
      n152 = Close Reference(reference=w327, error in (no error)=w338) -> (error out=w360:errorcluster)
      n153 = call <resource>:"GDSError_ReportError.vi"("error in (no error)"=w360) -> ("error out"=w332:errorcluster)  [unwired: 18 in]
      n154 = call-dynamic "Destroy.vi"("ClassWriter.lvclass"=w330, "error in (no error)"=w332) -> ()  [unwired: 17 in, 1 out]
    }
    frame "UpdateMessageClasses" {
      w406 = refnum<vi> refnum  # LVClassLibrary
      # "From Message Class Ref\nGet Actor method"
      n155 = call <resource>:"mxLvGetItemRef.vi"("Item"=w381) -> ("Item Refnum"=w405:refnum<vi>, "error out"=w386:errorcluster)  [unwired: 1 in, 1 out]
      n156 = To More Specific Class(target class=w406, reference=w405, error in=w386) -> (specific class reference=w380:refnum<vi>, error out=w385:errorcluster)
      n157 = call-dynamic "Init.vi"("ClassWriter in"=refnum<class "ClassWriter.lvclass"> refnum, "error in (no error)"=w385) -> ("ClassWriter out"=w388:refnum<class "ClassWriter.lvclass">, "error out"=w390:errorcluster)  [unwired: 16 in]
      n158 = call <resource>:"GdsLanguage_GetTranslatedString.vi"("StringID(s)"="UpdateMessageClass" ("Message(Exit)"), "error in (no error)"=w390) -> ("FirstStringOut"=w391:string, "error out"=w389:errorcluster)  [unwired: 14 in, 2 out]
      n159 = disable-structure shown="Enabled" {
        disable-tunnel: w391 -> [w411 _]
        disable-tunnel: [w410 w413] -> w379
        disable-tunnel: w389 -> [w409 w413]
        disable-tunnel: w388 -> [w408 w412]
        disable-tunnel: [w407 w412] -> w382
        frame Enabled {
          n160 = call-dynamic "ProgressWindow.vi"("ClassWriter in"=w408, "Message(Exit)"=w411, "error in (no error)"=w409) -> ("ClassWriter out"=w407:refnum<class "ClassWriter.lvclass">, "error out"=w410:errorcluster)  [unwired: 15 in]
        }
        frame Disabled {
        }
      }
      n161 = property class="LVClassLibrary"(reference=w380, error in=w379) -> (reference out=w398:refnum<vi>, error out=w403:errorcluster, "Project"=w404:refnum<vi>)
      n162 = property class="Project"(reference=w404, error in=w403) -> (reference out=w399:refnum<vi>, error out=w400:errorcluster, "App Ref"=w402:refnum<vi>)
      n163 = invoke class="LVClassLibrary" method="Get All Descendents"(reference=w398, error in=w400, "Type"="VI") -> (reference out=w395:refnum<vi>, error out=w396:errorcluster, "All Descendents"=w393:refnum<vi>[])  [unwired: 4 in, 4 out]
      n164 = for {
        tunnel: w402 -> [w421]
        shift-right: [w415] -> w394
        shift-left: w396 -> [w418]
        tunnel: w393 -> [w419] mode=indexing
        tunnel: w395 -> [w420]
        tunnel: w380 -> [w414]
        stop <- w415 stop-if-true
        n165 = invoke class="LVClassLibrary" method="Get Source Scope"(reference=w420, error in=w418, "SourceRef"=w419) -> (error out=w417:errorcluster, "GetSourceScope"=w416:T15)  [unwired: 2 in, 3 out]
        n166 = case shown="\"public\", Default" w416 {
          tunnel: [w422 w430] -> w415
          tunnel: w421 -> [_ w429]
          tunnel: w419 -> [_ w426]
          tunnel: w417 -> [w422 w425]
          tunnel: w414 -> [_ w423]
          frame "private", "protected" {
          }
          frame "public", Default {
            n167 = property class="ProjectItem"(reference=w426, error in=w425) -> (error out=w427:errorcluster, "Path"=w428:path)  [unwired: 1 out]
            n168 = call <resource>:"MM.vi"("AppInst"=w429, "ActorMethod"=w428, "ActorClassItemRef(Don't Delete)"=w423, "OnlyUpdate(if needed,False)"=FALSE, "error in"=w427) -> ("error out"=w430:errorcluster)  [unwired: 14 in]
          }
        }
      }
      n169 = Close Reference(reference=w393, error in (no error)=w394) -> ()  [unwired: 1 out]
      n170 = Close Reference(reference=w402, error in (no error)=w394) -> (error out=w401:errorcluster)
      n171 = Close Reference(reference=w399, error in (no error)=w401) -> (error out=w384:errorcluster)
      n172 = call-dynamic "Destroy.vi"("ClassWriter.lvclass"=w382, "error in (no error)"=w384) -> ("error out"=w383:errorcluster)  [unwired: 17 in]
      n173 = call <resource>:"GDSError_ReportError.vi"("error in (no error)"=w383) -> ()  [unwired: 18 in, 1 out]
    }
    frame Default {
      n174 = Match Pattern(string=w433, regular expression="\\2E[Pp][Nn][Gg]") -> (before substring=w431:string, offset past match=w432:i32)  [unwired: 1 in, 2 out]
      n175 = case shown="Default" w432 {
        tunnel: w434 -> [w436 _]
        tunnel: w433 -> [_ _]
        tunnel: w431 -> [w437 _]
        frame Default {
          w443 = refnum<vi> refnum  # LVClassLibrary
          n176 = call <resource>:"mxLvGetItemRef.vi"("Item"=w436) -> ("Item Refnum"=w442:refnum<vi>, "error out"=w441:errorcluster)  [unwired: 1 in, 1 out]
          n177 = call <resource>:"GOOP_ApplyOverlayIcon.vi"("error in (no error)"=w441, "IconName(NoPngExtension)"=w437, "Object"=w436) -> ("error out"=w440:errorcluster)  [unwired: 8 in]
          n178 = To More Specific Class(target class=w443, reference=w442) -> (specific class reference=w439:refnum<vi>)  [unwired: 1 in, 1 out]
          n179 = call <resource>:"GDSLvClass_StoreClassItemIcon.vi"("Library Refnum"=w439, "ClassItemIconName"=w437, "error in (no error)"=w440) -> ("error out"=w438:errorcluster)  [unwired: 15 in, 1 out]
          n180 = Close Reference(reference=w439, error in (no error)=w438) -> ()  [unwired: 1 out]
        }
        frame -1 {
        }
      }
    }
    frame "ModifyInheritance" {
      w458 = refnum<vi> refnum  # LVClassLibrary
      # "Not allowed"
      n181 = call <resource>:"GOOP_GetClassProvider.vi"("New Item Parent/Object"=w463, "ProviderClassType"=GOOP_ClassProviderClassType."ClassWriter") -> ("ProjectItem"=w459:refnum<vi>, "LVClass.Open"=w450:refnum<vi>, "error out"=w449:errorcluster)  [unwired: 15 in]
      n182 = To More Specific Class(target class=w458, reference=w459) -> (specific class reference=w444:refnum<vi>)  [unwired: 1 in, 1 out]
      n183 = call <resource>:"GOOP_GetDefaultInstance.vi"("error in"=w449, "LVClassIn"=w450) -> ("error out"=w445:errorcluster, "ClassWriter.lvclass"=w448:refnum<class "ClassWriter.lvclass">, "LVClassOut"=w451:refnum<vi>)  [unwired: 7 in]
      n184 = call-dynamic "Init.vi"("ClassWriter in"=w448, "error in (no error)"=w445, "LVClassLibrary Refnum"=w444) -> ("ClassWriter out"=w447:refnum<class "ClassWriter.lvclass">, "error out"=w446:errorcluster)  [unwired: 15 in]
      n185 = call-dynamic "ChangeInheritanceDialog.vi"("ClassWriter in"=w447, "LvClass"=w444, "error in (no error)"=w446) -> ("ClassWriter out"=w456:refnum<class "ClassWriter.lvclass">, "BaseClassPath"=w452:path, "Cancelled"=w453:bool, "error out"=w455:errorcluster)  [unwired: 13 in]
      n186 = case shown="False" w453 {
        tunnel: w456 -> [w465 _]
        tunnel: w455 -> [w467 w474]
        tunnel: [w473 w474] -> w454
        tunnel: w444 -> [w472 _]
        tunnel: w452 -> [w471 _]
        frame False {
          n187 = call <resource>:"GdsLanguage_GetTranslatedString.vi"("StringID(s)"="ChangeingInheritanceStatusMessage" ("Message(Exit)"), "error in (no error)"=w467) -> ("FirstStringOut"=w468:string, "error out"=w469:errorcluster)  [unwired: 14 in, 2 out]
          n188 = call-dynamic "ProgressWindow.vi"("ClassWriter in"=w465, "Message(Exit)"=w468, "error in (no error)"=w469) -> ("ClassWriter out"=w464:refnum<class "ClassWriter.lvclass">, "error out"=w466:errorcluster)  [unwired: 15 in]
          n189 = call-dynamic "ChangeInheritance.vi"("ClassWriter in"=w464, "LvClass"=w472, "NewBaseClass(Empty=ConvertClassToBaseClass)"=w471, "error in (no error)"=w466) -> ("error out"=w473:errorcluster)  [unwired: 14 in, 1 out]
        }
        frame True {
        }
      }
      n190 = call-dynamic "Destroy.vi"("ClassWriter.lvclass"=w447, "error in (no error)"=w454) -> ("error out"=w457:errorcluster)  [unwired: 17 in]
      n191 = Close Reference(reference=w451, error in (no error)=w457) -> (error out=w462:errorcluster)
      n192 = Close Reference(reference=w444, error in (no error)=w462) -> (error out=w461:errorcluster)
      n193 = call <resource>:"GDSError_ReportError.vi"("error in (no error)"=w461) -> ()  [unwired: 18 in, 1 out]
    }
    frame "UmlViewClass" {
      # "OK to do"
      n194 = call <resource>:"mxLvGetItemRef.vi"("Item"=w480) -> ("Item Refnum"=w502:refnum<vi>, "error out"=w492:errorcluster)  [unwired: 1 in, 1 out]
      n195 = property class="ProjectItem"(reference=w502, error in=w492) -> (reference out=w496:refnum<vi>, error out=w475:errorcluster, "Project"=w501:refnum<vi>, "Type String"=w494:string, "Target"=w479:refnum<vi>)
      n196 = case shown="Default" w494 {
        tunnel: w496 -> [w504 w510 w516]
        tunnel: [w504 w506 w512] -> w495
        tunnel: [_ w505 w511] -> w493
        frame Default {
        }
        frame "LvClass" {
          w509 = refnum<vi> refnum  # LVClassLibrary
          n197 = To More Specific Class(target class=w509, reference=w510) -> (specific class reference=w508:refnum<vi>, error out=w507:errorcluster)  [unwired: 1 in]
          n198 = property class="LVClassLibrary"(reference=w508, error in=w507) -> (reference out=w506:refnum<vi>, "Path"=w505:path)  [unwired: 1 out]
        }
        frame "VI" {
          w515 = refnum<vi> refnum  # ProjectItem
          n199 = To More Specific Class(target class=w515, reference=w516) -> (specific class reference=w514:refnum<vi>, error out=w513:errorcluster)  [unwired: 1 in]
          n200 = property class="ProjectItem"(reference=w514, error in=w513) -> (reference out=w512:refnum<vi>, "Path"=w511:path)  [unwired: 1 out]
        }
      }
      n201 = property class="TargetItem"(reference=w479, error in=w475) -> (reference out=w477:refnum<vi>, error out=w476:errorcluster, "Name"=w478:string)
      n202 = property class="Project"(reference=w501, error in=w475) -> (reference out=w498:refnum<vi>, error out=w499:errorcluster, "Name"=w500:string)
      n203 = Close Reference(reference=w477, error in (no error)=w476) -> ()  [unwired: 1 out]
      n204 = Close Reference(reference=w498, error in (no error)=w499) -> (error out=w497:errorcluster)
      n205 = Close Reference(reference=w495, error in (no error)=w497) -> (error out=w488:errorcluster)
      n206 = call-dynamic "Init.vi"("ClassWriter in"=refnum<class "ClassWriter.lvclass"> refnum, "error in (no error)"=w488) -> ("ClassWriter out"=w483:refnum<class "ClassWriter.lvclass">, "error out"=w487:errorcluster)  [unwired: 16 in]
      n207 = call <resource>:"GdsLanguage_GetTranslatedString.vi"("StringID(s)"="UmlViewClasses" ("Message(Exit)"), "error in (no error)"=w487) -> ("FirstStringOut"=w491:string, "error out"=w490:errorcluster)  [unwired: 14 in, 2 out]
      n208 = call-dynamic "ProgressWindow.vi"("ClassWriter in"=w483, "Message(Exit)"=w491, "error in (no error)"=w490) -> ("ClassWriter out"=w484:refnum<class "ClassWriter.lvclass">, "error out"=w486:errorcluster)  [unwired: 15 in]
      n209 = call <resource>:"GOOP_UMLEditor_CallMain.vi"("Enum"=GOOP_UMLEditor_CallMainAction."ReverseEngineering:OneClass", "Project"=w500, "Class/VI-Path"=w493, "Target"=w478, "error in (no error)"=w486) -> ("error out"=w485:errorcluster)  [unwired: 14 in]
      n210 = call-dynamic "Destroy.vi"("ClassWriter.lvclass"=w484, "error in (no error)"=w485) -> ("error out"=w482:errorcluster)  [unwired: 17 in]
      n211 = call <resource>:"GDSError_ReportError.vi"("error in (no error)"=w482) -> ()  [unwired: 18 in, 1 out]
    }
    frame "GoopEditClassApperance" {
      w529 = refnum<vi> refnum  # LVClassLibrary
      # "Not allowed"
      n212 = call <resource>:"mxLvGetItemRef.vi"("Item"=w527) -> ("Item"=w525:T16, "Item Refnum"=w528:refnum<vi>, "error out"=w519:errorcluster)  [unwired: 1 in]
      n213 = To More Specific Class(target class=w529, reference=w528) -> (specific class reference=w517:refnum<vi>)  [unwired: 1 in, 1 out]
      n214 = call <resource>:"GOOP_CheckClassState.vi"("error in"=w519, "Library Refnum"=w517) -> ("error out"=w518:errorcluster)  [unwired: 9 in]
      n215 = call <resource>:"BaseProvider_Configuration.vi"("ClassRef/ClassPath(If empty Configuration default will be modified)"=w517, "Error In"=w518) -> ("Error Out"=w524:errorcluster)  [unwired: 17 in]
      n216 = call <resource>:"GDSLvClass_ReadClassColors.vi"("Library Refnum"=w517, "error in (no error)"=w524) -> ("Library Refnum"=w521:refnum<vi>, "ClassItemIconName(NoExtension)"=w526:string, "error out"=w523:errorcluster)  [unwired: 12 in, 3 out]
      n217 = call <resource>:"GOOP_ApplyOverlayIcon.vi"("error in (no error)"=w523, "IconName(NoPngExtension)"=w526, "Object"=w525) -> ("error out"=w522:errorcluster)  [unwired: 8 in]
      n218 = Close Reference(reference=w521, error in (no error)=w522) -> (error out=w520:errorcluster)
      n219 = call <resource>:"GDSError_ReportError.vi"("error in (no error)"=w520) -> ()  [unwired: 18 in, 1 out]
    }
  }
